vi "valueToString.vi"(8 "error in (no error)":errorcluster, 10 "Value Type in":T1 items=["ctBool"=0, "ctInt"=1, "ctFloat"=2, "ctString"=3, "ctList"=4, "ctDict"=5, "ctRatio"=6, "ctProc"=7, "ctObject"=8, "ctBinaryData"=9, "ctFunc"=10, "ctComplexNumber"=11, "ctStruct"=12, "ctEnumeration"=13, "ctUndefined"=65535], 11 "Value in":refnum<class "IBaseObject.lvclass">) -> (0 "error out":errorcluster, 2 "String out":string, 3 "Value out":refnum<class "IBaseObject.lvclass">)   [LabVIEW 2022 SP3, in "Property Editor.lvlib"]
uses:
  Property Editor.lvlib
  Public/Classes/daqCoreTypes/IBoolean/IBoolean.lvclass
  Public/Classes/IBaseObject/IBaseObject.lvclass
  Public/Classes/IBaseObject/Polymorphic/borrowInterface/borrowBooleanInterface.vi
  Public/Classes/IBaseObject/Polymorphic/borrowInterface/borrowIntegerInterface.vi
  Public/Classes/daqCoreTypes/IInteger/IInteger.lvclass
  Public/Classes/IBaseObject/Polymorphic/borrowInterface/borrowFloatInterface.vi
  Public/Classes/daqCoreTypes/IFloat/IFloat.lvclass
  Public/Classes/IBaseObject/Polymorphic/borrowInterface/borrowStringInterface.vi
  Public/Classes/daqCoreTypes/IString/IString.lvclass
  Public/Classes/IBaseObject/Polymorphic/borrowInterface/borrowRatioInterface.vi
  Public/Classes/daqCoreTypes/IRatio/IRatio.lvclass
  Public/Classes/IBaseObject/Polymorphic/borrowInterface/borrowComplexNumberInterface.vi
  Public/Classes/daqCoreTypes/IComplexNumber/IComplexNumber.lvclass
  Public/Classes/daqCoreTypes/IEnumeration/IEnumeration.lvclass
  Public/Classes/IBaseObject/Polymorphic/borrowInterface/borrowEnumerationInterface.vi
  Public/Classes/daqCoreTypes/IEnumerationType/IEnumerationType.lvclass
  Public/TypeDef/CoreType.ctl
  openDAQ.lvlib
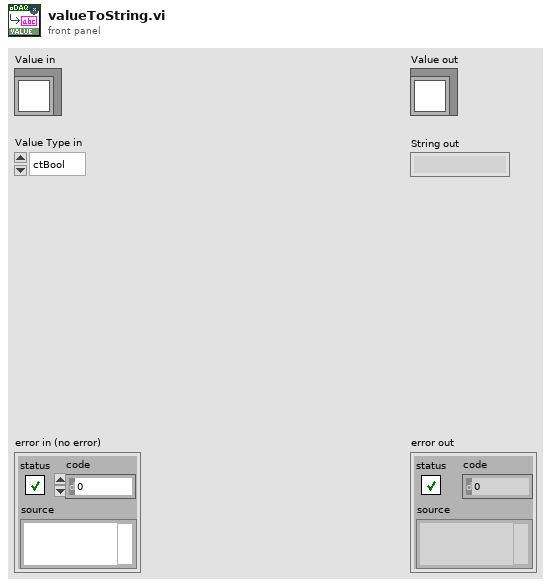
[diagram p1: front panel]
types:
  T1 = typedef "openDAQ.lvlib/CoreType.ctl" = u16
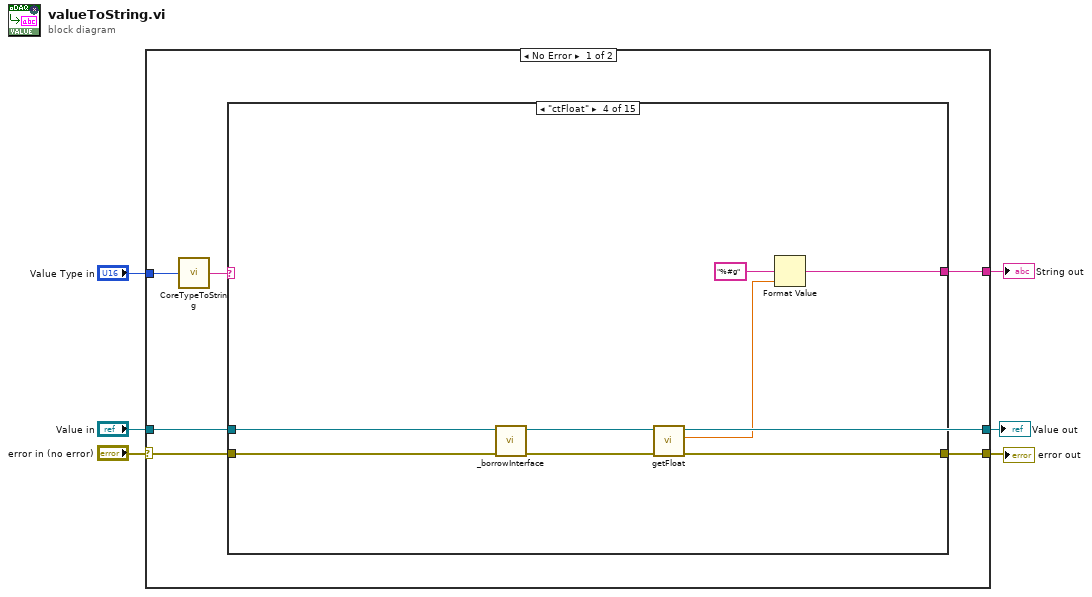
[diagram p0: block diagram]
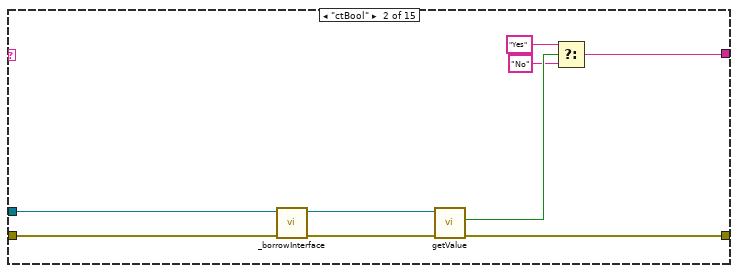
[diagram p3: hidden frame]
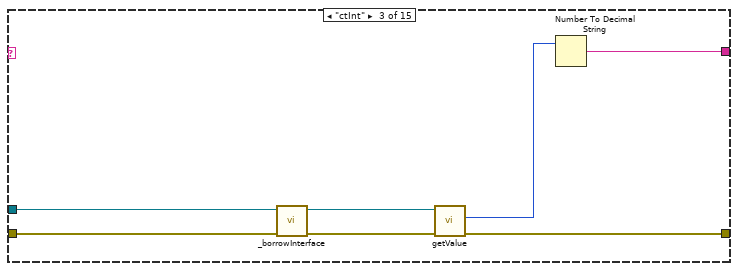
[diagram p4: hidden frame]
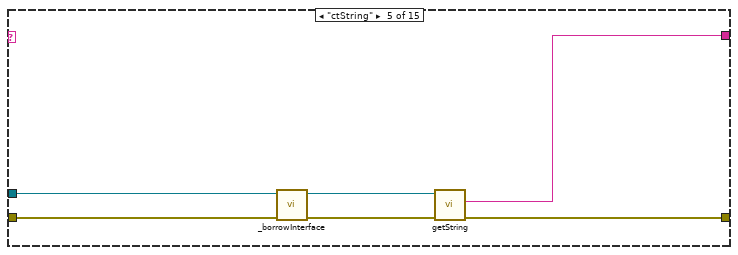
[diagram p5: hidden frame]
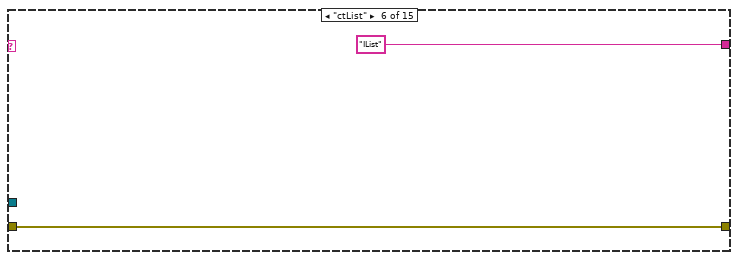
[diagram p6: hidden frame]
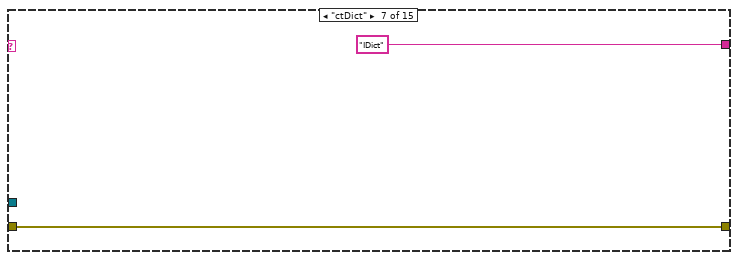
[diagram p7: hidden frame]
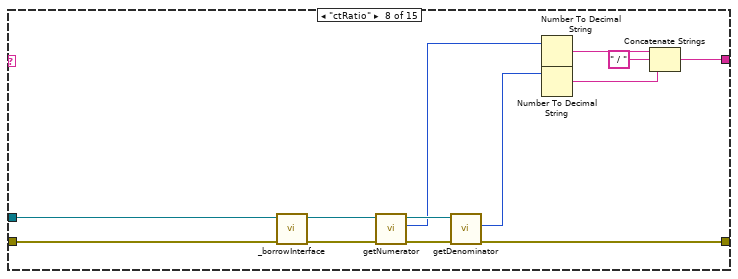
[diagram p8: hidden frame]
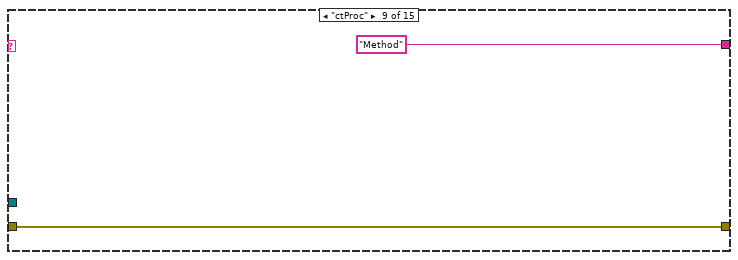
[diagram p9: hidden frame]
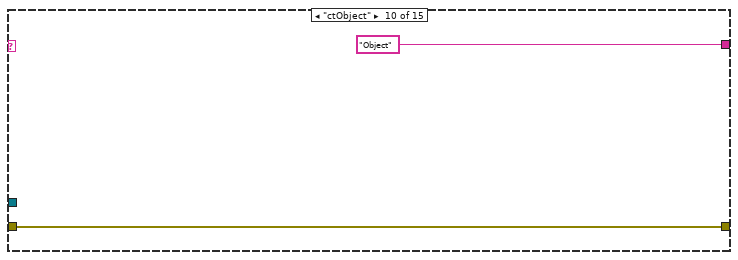
[diagram p10: hidden frame]
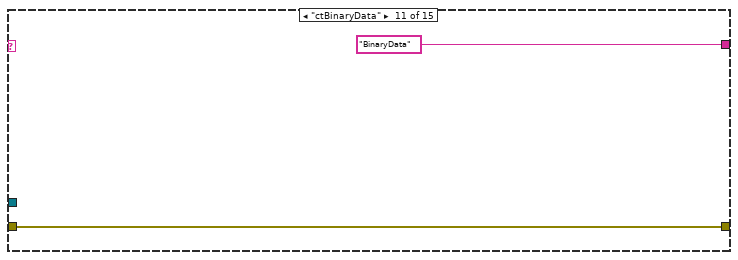
[diagram p11: hidden frame]
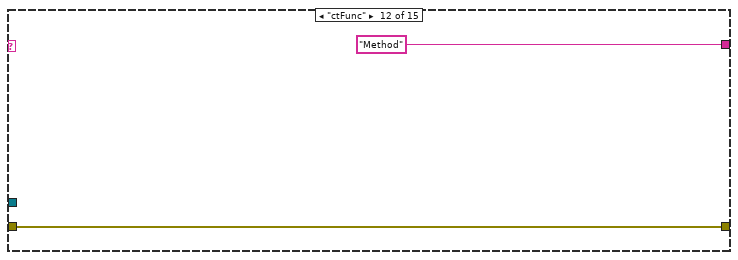
[diagram p12: hidden frame]
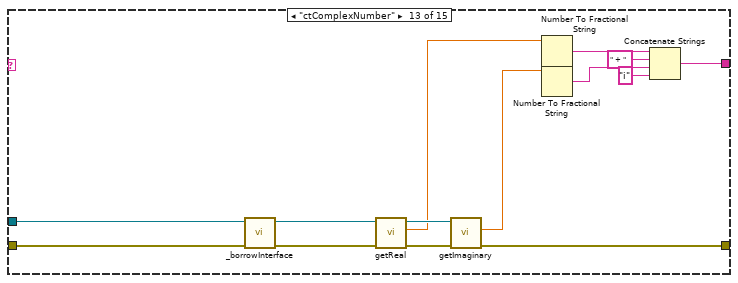
[diagram p13: hidden frame]
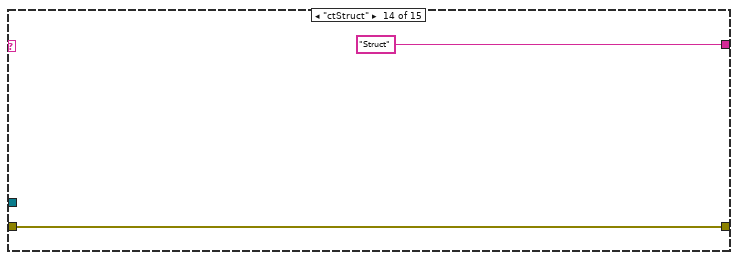
[diagram p14: hidden frame]
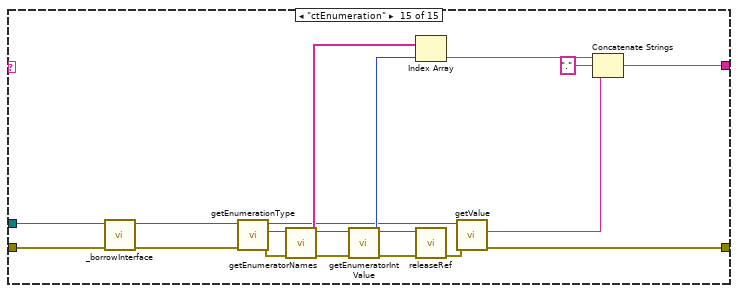
[diagram p15: hidden frame]
diagram:
  n1 = case shown="No Error" "error in (no error)" {
    selector: "error in (no error)" -> [w10 w105]
    tunnel: [w9 w105] -> w6
    tunnel: "Value Type in" -> [w12 _]
    tunnel: "Value in" -> [w7 w104]
    tunnel: [w8 _] -> w2
    tunnel: [w7 w104] -> w1
    frame No Error {
      n2 = call "CoreTypeToString.vi"("Value Type out"=w12) -> ("String"=w11:string)  [unwired: 4 in]
      n3 = case shown="\"ctFloat\"" w11 {
        tunnel: w7 -> [_ w22 w29 w37 w43 _ _ w60 _ _ _ _ w82 _ w103]
        tunnel: w10 -> [w13 w21 w28 w36 w42 w45 w47 w59 w62 w64 w66 w68 w81 w84 w102]
        tunnel: [w13 w17 w25 w33 w39 w45 w47 w52 w62 w64 w66 w68 w74 w84 w89] -> w9
        tunnel: [_ w14 w24 w32 w38 "IList" "IDict" w50 "Method" "Object" "BinaryData" "Method" w72 "Struct" w85] -> w8
        frame Default {
        }
        frame "ctBool" {
          n4 = call-poly "_borrowInterface.vi"("error in (no error)"=w21, "IBaseObject in"=w22) -> ("error out"=w19:errorcluster, "Bool out"=w20:refnum<class "IBoolean.lvclass">)  [unwired: 6 in, 2 out]
          n5 = call "getValue.vi"("error in (no error)"=w19, "IBoolean in"=w20) -> ("error out"=w17:errorcluster, "Value out"=w18:bool)  [unwired: 7 in, 1 out]
          n6 = Select(t="Yes", s=w18, f="No") -> (s? t:f=w14:string)
        }
        frame "ctInt" {
          n7 = call-poly "_borrowInterface.vi"("error in (no error)"=w28, "IBaseObject in"=w29) -> ("error out"=w26:errorcluster, "Integer out"=w27:refnum<class "IInteger.lvclass">)  [unwired: 6 in, 2 out]
          n8 = call "getValue.vi"("error in (no error)"=w26, "IInteger in"=w27) -> ("error out"=w25:errorcluster, "Value out"=w23:i32)  [unwired: 7 in, 1 out]
          n9 = Number To Decimal String(number=w23) -> (decimal integer string=w24:string)  [unwired: 1 in]
        }
        frame "ctFloat" {
          n10 = call-poly "_borrowInterface.vi"("error in (no error)"=w36, "IBaseObject in"=w37) -> ("error out"=w34:errorcluster, "Float out"=w35:refnum<class "IFloat.lvclass">)  [unwired: 6 in, 2 out]
          n11 = call "getFloat.vi"("error in (no error)"=w34, "IFloat in"=w35) -> ("error out"=w33:errorcluster, "float"=w31:dbl)  [unwired: 7 in, 1 out]
          n12 = Format Value(format string="%#g", value (0)=w31) -> (output string=w32:string)  [unwired: 1 in]
        }
        frame "ctString" {
          n13 = call-poly "_borrowInterface.vi"("error in (no error)"=w42, "IBaseObject in"=w43) -> ("error out"=w40:errorcluster, "String out"=w41:refnum<class "IString.lvclass">)  [unwired: 6 in, 2 out]
          n14 = call "getString.vi"("error in (no error)"=w40, "IString in"=w41) -> ("error out"=w39:errorcluster, "String out"=w38:string)  [unwired: 7 in, 1 out]
        }
        frame "ctList" {
        }
        frame "ctDict" {
        }
        frame "ctRatio" {
          n15 = call-poly "_borrowInterface.vi"("error in (no error)"=w59, "IBaseObject in"=w60) -> ("error out"=w57:errorcluster, "Ratio out"=w58:refnum<class "IRatio.lvclass">)  [unwired: 6 in, 2 out]
          n16 = call "getNumerator.vi"("error in (no error)"=w57, "IRatio in"=w58) -> ("error out"=w56:errorcluster, "Numerator out"=w54:i64, "IRatio out"=w55:refnum<class "IRatio.lvclass">)  [unwired: 7 in]
          n17 = call "getDenominator.vi"("error in (no error)"=w56, "IRatio in"=w55) -> ("error out"=w52:errorcluster, "Denominator out"=w53:i64)  [unwired: 7 in, 1 out]
          n18 = Number To Decimal String(number=w54) -> (decimal integer string=w49:string)  [unwired: 1 in]
          n19 = Number To Decimal String(number=w53) -> (decimal integer string=w48:string)  [unwired: 1 in]
          n20 = Concatenate Strings(w49, " / ", w48) -> (w50:string)
        }
        frame "ctProc" {
        }
        frame "ctObject" {
        }
        frame "ctBinaryData" {
        }
        frame "ctFunc" {
        }
        frame "ctComplexNumber" {
          n21 = call-poly "_borrowInterface.vi"("error in (no error)"=w81, "IBaseObject in"=w82) -> ("error out"=w79:errorcluster, "ComplexNumber out"=w80:refnum<class "IComplexNumber.lvclass">)  [unwired: 6 in, 2 out]
          n22 = call "getReal.vi"("error in (no error)"=w79, "IComplexNumber in"=w80) -> ("error out"=w78:errorcluster, "Complex Real out"=w76:dbl, "IComplexNumber out"=w77:refnum<class "IComplexNumber.lvclass">)  [unwired: 7 in]
          n23 = call "getImaginary.vi"("error in (no error)"=w78, "IComplexNumber in"=w77) -> ("error out"=w74:errorcluster, "Complex Imaginary out"=w75:dbl)  [unwired: 7 in, 1 out]
          n24 = Number To Fractional String(number=w76) -> (F-format string=w71:string)  [unwired: 3 in]
          n25 = Number To Fractional String(number=w75) -> (F-format string=w70:string)  [unwired: 3 in]
          n26 = Concatenate Strings(w71, " + ", w70, "i") -> (w72:string)
        }
        frame "ctStruct" {
        }
        frame "ctEnumeration" {
          n27 = call-poly "_borrowInterface.vi"("error in (no error)"=w102, "IBaseObject in"=w103) -> ("error out"=w92:errorcluster, "Enumeration out"=w93:refnum<class "IEnumeration.lvclass">)  [unwired: 6 in, 2 out]
          n28 = call "getEnumerationType.vi"("error in (no error)"=w92, "IEnumeration in"=w93) -> ("error out"=w99:errorcluster, "Enumeration Type out"=w101:refnum<class "IEnumerationType.lvclass">, "IEnumeration out"=w91:refnum<class "IEnumeration.lvclass">)  [unwired: 7 in]
          n29 = call "getEnumeratorNames.vi"("error in (no error)"=w99, "IEnumerationType in"=w101) -> ("error out"=w98:errorcluster, "Enumerator Names out"=w95:string[], "IEnumerationType out"=w100:refnum<class "IEnumerationType.lvclass">)  [unwired: 7 in]
          n30 = call "getEnumeratorIntValue.vi"("error in (no error)"=w98, "IEnumerationType in"=w100) -> ("error out"=w96:errorcluster, "Int Value out"=w94:i64, "IEnumerationType out"=w97:refnum<class "IEnumerationType.lvclass">)  [unwired: 7 in]
          n31 = Index Array(array=w95, index=w94) -> (element=w87:string)
          n32 = call-dynamic "releaseRef.vi"("error in (no error)"=w96, "IBaseObject in"=w97) -> ("error out"=w90:errorcluster)  [unwired: 9 in]
          n33 = call "getValue.vi"("error in (no error)"=w90, "Enumeration in"=w91) -> ("error out"=w89:errorcluster, "Value out"=w86:string)  [unwired: 7 in, 1 out]
          n34 = Concatenate Strings(w87, ".", w86) -> (w85:string)
        }
      }
    }
    frame Error {
    }
  }
  "error out" <- w6
  "String out" <- w2
  "Value out" <- w1
